vi "ingest.mcap_free.vi"(8 "error in":errorcluster, 11 "McapIngestStaging in":refnum<class "McapIngestStaging.lvclass">) -> (0 "error out":errorcluster, 3 "McapIngestStaging out":refnum<class "McapIngestStaging.lvclass">)   [LabVIEW 2020, in "McapIngestStaging.lvclass"]
doc: "Releases the handle and its associated resources."
uses:
  McapIngestStaging.lvclass
  McapIngestStaging.lvclass/McapIngestStaging.ctl
  client.lvlib
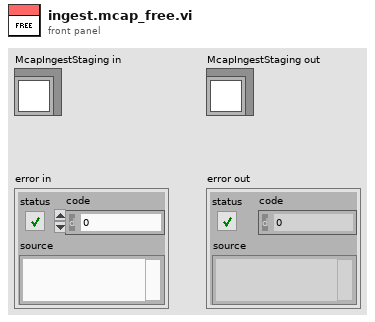
[diagram p1: front panel]
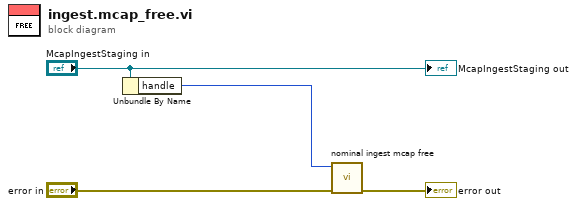
[diagram p0: block diagram]
diagram:
  n1 = Unbundle By Name("McapIngestStaging in") -> ("handle"=w2:i32)
  n2 = call "nominal ingest mcap free.vi"("error in (no error)"="error in", "staging"=w2) -> ("error out"=→"error out":errorcluster)  [unwired: 8 in, 1 out]
  "McapIngestStaging out" <- "McapIngestStaging in"
